vi "Build_Full_Address.vi"(7 "Version (no version)":string, 8 "error in (no error)":errorcluster, 9 "API Root":string, 10 "Port (protocol specific)":u16, 11 "Base URL":string) -> (0 "error out":errorcluster, 2 "Full URL":string)   [LabVIEW 2019, in "ByteREST.lvlib" / "RESTBase.lvclass"]
uses:
  RESTBase.lvclass
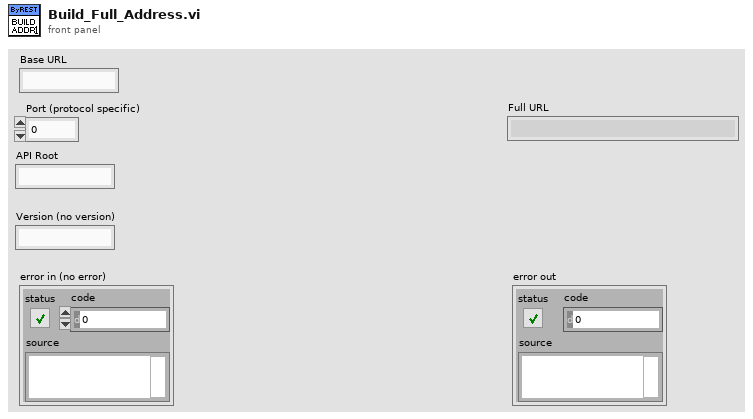
[diagram p1: front panel]
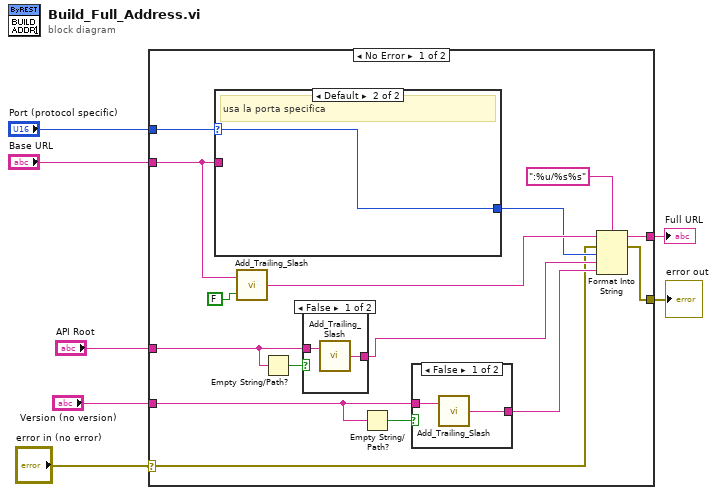
[diagram p0: block diagram]
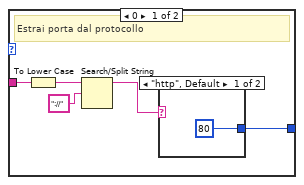
[diagram p4: hidden frame]
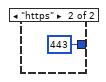
[diagram p5: hidden frame]
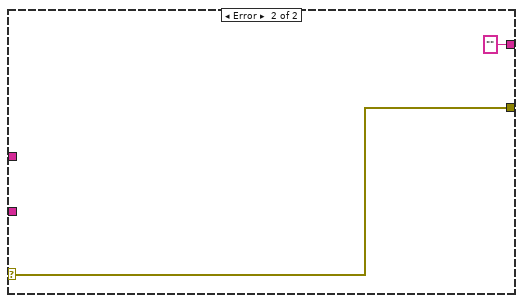
[diagram p6: hidden frame]
diagram:
  n1 = case shown="No Error" "error in (no error)" {
    selector: "error in (no error)" -> [w8 w38]
    tunnel: "Port (protocol specific)" -> [w22 _]
    tunnel: "Base URL" -> [w21 _]
    tunnel: [w20 ""] -> w5
    tunnel: "API Root" -> [w15 _]
    tunnel: "Version (no version)" -> [w12 _]
    tunnel: [w9 w38] -> w2
    frame No Error {
      n2 = case shown="Default" w22 {
        selector: w22 -> [_ w36]
        tunnel: w21 -> [w31 _]
        tunnel: [w29 w36] -> w16
        frame 0 {
          # "Estrai porta dal protocollo"
          n3 = To Lower Case(string=w31) -> (all lower case string=w30:string)
          n4 = Search/Split String(string=w30, search string/char (-)="://") -> (substring before match=w32:string)  [unwired: 1 in, 2 out]
          n5 = case shown="\"http\", Default" w32 {
            tunnel: [80 443] -> w29
            frame "http", Default {
            }
            frame "https" {
            }
          }
        }
        frame Default {
          # "usa la porta specifica"
        }
      }
      n6 = call "Add_Trailing_Slash.vi"("Wanted? (True)"=FALSE, "path"=w21) -> ("path with trailing slash"=w19:string)
      n7 = Empty String/Path?(string/path=w15) -> (empty?=w14:bool)
      n8 = case shown="False" w14 {
        tunnel: w15 -> [w27 w28]
        tunnel: [w26 w28] -> w10
        frame False {
          n9 = call "Add_Trailing_Slash.vi"("path"=w27) -> ("path with trailing slash"=w26:string)  [unwired: 1 in]
        }
        frame True {
        }
      }
      n10 = Empty String/Path?(string/path=w12) -> (empty?=w13:bool)
      n11 = case shown="False" w13 {
        tunnel: w12 -> [w24 w25]
        tunnel: [w23 w25] -> w11
        frame False {
          n12 = call "Add_Trailing_Slash.vi"("path"=w24) -> ("path with trailing slash"=w23:string)  [unwired: 1 in]
        }
        frame True {
        }
      }
      n13 = Format Into String(format string=":%u/%s%s", initial string=w19, error in=w8, w16, w10, w11) -> (resulting string=w20:string, error out=w9:errorcluster)
    }
    frame Error {
    }
  }
  "Full URL" <- w5
  "error out" <- w2
